vi "SPD.Insens Meas Insens_Grid.vi"(5 "Continue":refnum<vi>, 6 "deadtime index":i32, 7 "Progress":refnum<vi>, 8 "Error In":errorcluster, 11 "SPD.Stand Ctrl in":T2={"spdDeviceSession"={"spdRef"=0, "connected"=FALSE, "spdName"="", "specification"={"diod case"=enum."default", "type"=enum."Unknown", "frequency"=enum."Unknown"}, "hidSPD.Controller"={"TSet"=0.0, "HV_bias"=0.0, "DDS_stb_code"=0}, "hidSPD.Sturtup Values"={"TSet"=0.0, "HV_bias"=0.0, "DDS_stb_code"=0}}, "DevBSession"={"DevBRef"="", "connected"=FALSE}, "FreqCSession"={"FreqCRef"="", "timeout"=0.0, "Gate"=0.0, "connected"=FALSE}, "8164BSession"={"Connection ID"=refnum, "Connected"=FALSE, "Info"="", "Slots Info"=[]}, "LeCroySession"={"LeCroySession"="", "connected"=FALSE}, "Events"={"DCRTest"=refnum, "Stop"=refnum}, "configFile"={"configFile ref"=refnum, "configFile path"=path "", "equipmentFile ref"=refnum}, "SPD.Meas Grid"={"DateTime"="", "DT"=[], "Insensitivity"=[], "Temprature"=[], "Stb_code"=[], "HV_Bias"=[]}, "SPD.Queues"={"state queue"=refnum}, "Console"=refnum} {"spdDeviceSession"."hidSPD.Sturtup Values"."HV_bias" format="%#_6p, V"; "spdDeviceSession"."hidSPD.Sturtup Values"."TSet" format="%#_6p, DegC"; "spdDeviceSession"."hidSPD.Controller"."HV_bias" format="%#_6p, V"; "spdDeviceSession"."hidSPD.Controller"."TSet" format="%#_6p, DegC"}) -> (0 "Error Out":errorcluster, 1 "pass":bool, 2 "Report":string, 3 "SPD.Stand Ctrl out":T2={"spdDeviceSession"={"spdRef"=0, "connected"=FALSE, "spdName"="", "specification"={"diod case"=enum."default", "type"=enum."Unknown", "frequency"=enum."Unknown"}, "hidSPD.Controller"={"TSet"=0.0, "HV_bias"=0.0, "DDS_stb_code"=0}, "hidSPD.Sturtup Values"={"TSet"=0.0, "HV_bias"=0.0, "DDS_stb_code"=0}}, "DevBSession"={"DevBRef"="", "connected"=FALSE}, "FreqCSession"={"FreqCRef"="", "timeout"=0.0, "Gate"=0.0, "connected"=FALSE}, "8164BSession"={"Connection ID"=refnum, "Connected"=FALSE, "Info"="", "Slots Info"=[]}, "LeCroySession"={"LeCroySession"="", "connected"=FALSE}, "Events"={"DCRTest"=refnum, "Stop"=refnum}, "configFile"={"configFile ref"=refnum, "configFile path"=path "", "equipmentFile ref"=refnum}, "SPD.Meas Grid"={"DateTime"="", "DT"=[], "Insensitivity"=[], "Temprature"=[], "Stb_code"=[], "HV_Bias"=[]}, "SPD.Queues"={"state queue"=refnum}, "Console"=refnum} {"spdDeviceSession"."hidSPD.Sturtup Values"."HV_bias" format="%#_6p, V"; "spdDeviceSession"."hidSPD.Sturtup Values"."TSet" format="%#_6p, DegC"; "spdDeviceSession"."hidSPD.Controller"."HV_bias" format="%#_6p, V"; "spdDeviceSession"."hidSPD.Controller"."TSet" format="%#_6p, DegC"})   [LabVIEW 2018]
uses:
  typedefs/SPD.Stand Ctrl.ctl
  Instruments/SPD HID Interface/hidSPDLibForLabView/LibVIs/hidSPD Controls/hidSPD Device Session.ctl
  Instruments/SPD HID Interface/hidSPDLibForLabView/LibVIs/hidSPD Controls/hidSPD.SPD specification.ctl
  Instruments/SPD HID Interface/hidSPDLibForLabView/LibVIs/hidSPD Controls/hidSPD SPD Diod Case.ctl
  Instruments/SPD HID Interface/hidSPDLibForLabView/LibVIs/hidSPD Controls/hidSPD SPD Type.ctl
  Instruments/SPD HID Interface/hidSPDLibForLabView/LibVIs/hidSPD Controls/hidSPD.STB Frequency.ctl
  Instruments/SPD HID Interface/hidSPDLibForLabView/LibVIs/hidSPD Controls/hidSPD Controller.ctl
  Instruments/KC705 DevBoard/typedefs/DevB.Session.ctl
  Instruments/KeySight 53230A/typedefs/FreqC.Session.ctl
  Instruments/KeySight 8164B/KeySight 8164B LAN InstrLib/typedefs/KeySight 8164B control.ctl
  Instruments/LeCroy SDA830/typedefs/LeCroy.Session.ctl
  typedefs/SPD.Events.ctl
  ConfigFile/SPD.Config File ctrl.ctl
  <vilib>/Utility/config.llb/Config Data RefNum.ctl
  typedefs/SPD.Meas Grid.ctl
  typedefs/SPD.Queues.ctl
  typedefs/SPD.Stand state.ctl
  typedefs/SPD.Common HW Setup ctr.ctl
  typedefs/SPD.QE Strobe_Phase Tune Limits.ctl
  <vilib>/Analysis/1siggen.llb/Ramp Pattern by Delta.vi
  <vilib>/Analysis/NI_AALBase.lvlib
  Instruments/KeySight 8164B/KeySight 8164B LAN InstrLib.lvlib
  <vilib>/Utility/config.llb/NI_LVConfig.lvlib
  Instruments/SPD HID Interface/hidSPDLibForLabView/hidSPDLibForLabView.lvlib
panel:
  out "XY Graph":T1(graph)
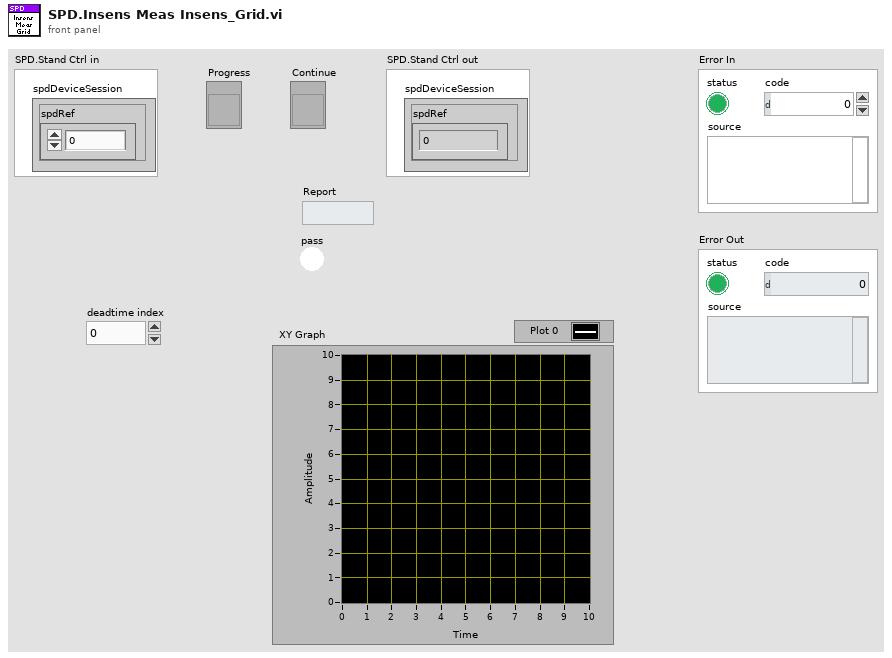
[diagram p1: front panel]
types:
  T1 = cluster{"result out":dbl[], "result out":dbl[]}[]
  T2 = typedef "SPD.Stand Ctrl.ctl" = cluster{"spdDeviceSession":T3, "DevBSession":T9, "FreqCSession":T10, "8164BSession":T11, "LeCroySession":T12, "Events":T13, "configFile":T14, "SPD.Meas Grid":T16, "SPD.Queues":T17, "Console":refnum<vi>}
  T3 = typedef "hidSPDLibForLabView.lvlib/hidSPD Device Session.ctl" = cluster{"spdRef":u64, "connected":bool, "spdName":string, "specification":T4, "hidSPD.Controller":T8, "hidSPD.Sturtup Values":T8}
  T4 = typedef "hidSPDLibForLabView.lvlib/hidSPD.SPD specification.ctl" = cluster{"diod case":T5, "type":T6, "frequency":T7}
  T5 = typedef "hidSPDLibForLabView.lvlib/hidSPD SPD Diod Case.ctl" = enum16{"Unknown", "default", "butterfly"}
  T6 = typedef "hidSPDLibForLabView.lvlib/hidSPD SPD Type.ctl" = enum16{"Unknown", "Free Run", "Gate"}
  T7 = typedef "hidSPDLibForLabView.lvlib/hidSPD.STB Frequency.ctl" = enum16{"Unknown", "312", "1250"}
  T8 = typedef "hidSPDLibForLabView.lvlib/hidSPD Controller.ctl" = cluster{"TSet":sgl, "HV_bias":sgl, "DDS_stb_code":u16}
  T9 = typedef "DevB.Session.ctl" = cluster{"DevBRef":refnum<visa-resource-name>, "connected":bool}
  T10 = typedef "FreqC.Session.ctl" = cluster{"FreqCRef":refnum<visa-resource-name>, "timeout":dbl, "Gate":dbl, "connected":bool}
  T11 = typedef "KeySight 8164B LAN InstrLib.lvlib/KeySight 8164B control.ctl" = cluster{"Connection ID":refnum<k5>, "Connected":bool, "Info":string, "Slots Info":string[]}
  T12 = typedef "LeCroy.Session.ctl" = cluster{"LeCroySession":refnum<visa-resource-name>, "connected":bool}
  T13 = typedef "SPD.Events.ctl" = cluster{"DCRTest":refnum<user-event>, "Stop":refnum<user-event>}
  T14 = typedef "SPD.Config File ctrl.ctl" = cluster{"configFile ref":T15, "configFile path":path, "equipmentFile ref":T15}
  T15 = typedef "NI_LVConfig.lvlib/Config Data RefNum.ctl" = refnum<k1>
  T16 = typedef "SPD.Meas Grid.ctl" = cluster{"DateTime":string, "DT":dbl[], "Insensitivity":dbl[], "Temprature":dbl[], "Stb_code":dbl[], "HV_Bias":dbl[][][][]}
  T17 = typedef "SPD.Queues.ctl" = cluster{"state queue":refnum<queue>}
  T18 = typedef "SPD.Common HW Setup ctr.ctl" = cluster{"FS":i32, "TS":i32, "Gate":dbl, "Att1 enable":bool, "Att3 enable":bool, "Att3 Att":dbl, "Scope setup file path":string, "Pset":dbl, "Set Pset":bool}
  T19 = typedef "SPD.DT&Insens Test Params.ctl" = cluster{"FS":i32, "TS":i32, "Att3":dbl, "Gate":dbl, "Num of Meas":i32, "ScopeRecallFile":string, "HistoSize":i32, "DT_min":u16, "DT_max":u16, "DT_step":u16, "Desired_DTs":dbl[], "Insens_bound":u16, "Insens_step":u16}
  T20 = typedef "SPD.QE Strobe_Phase Tune Limits.ctl" = cluster{"ph_start":i32, "ph_stop":i32, "ph_step":i32}
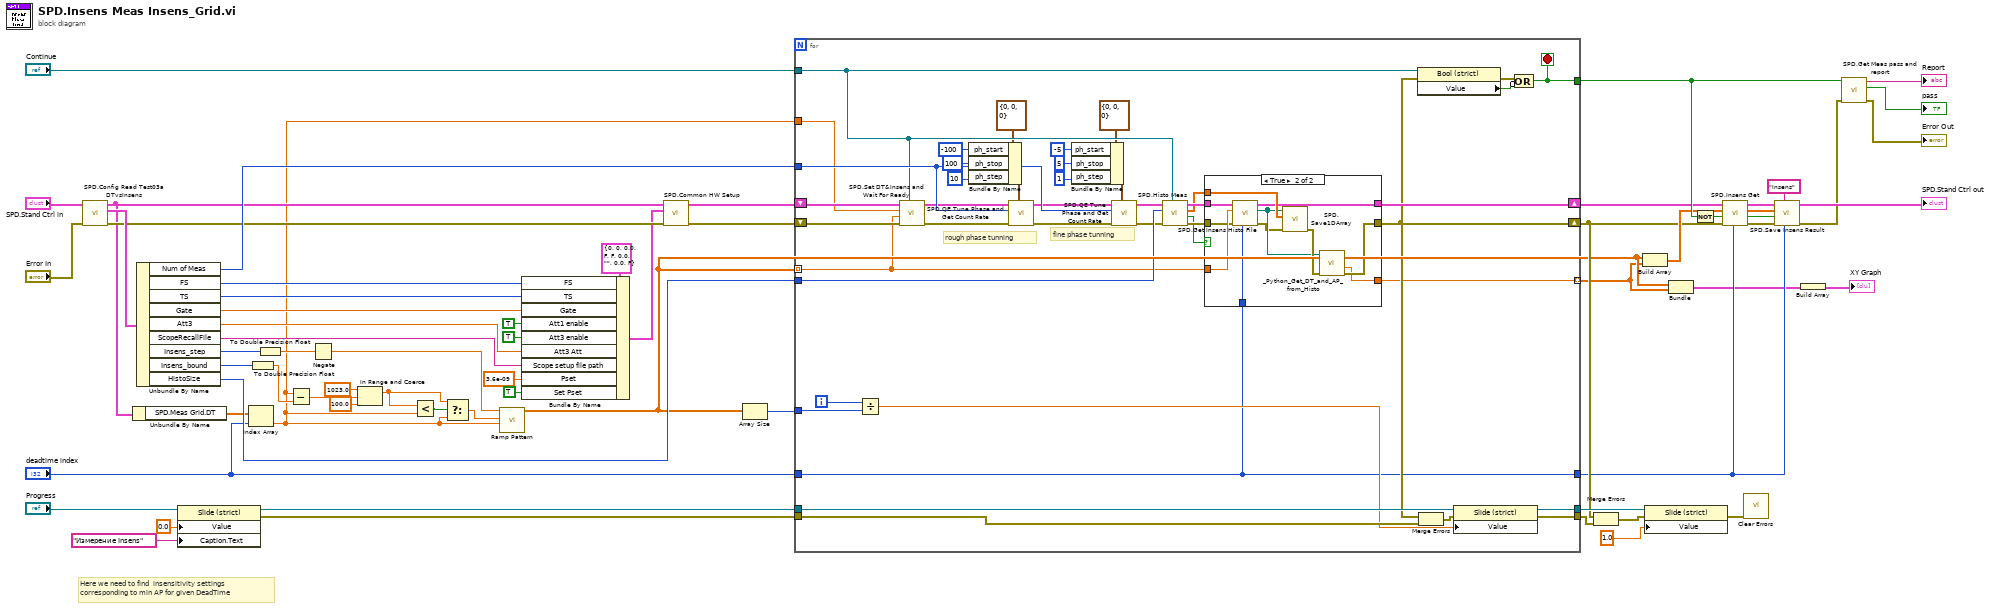
[diagram p0: block diagram]
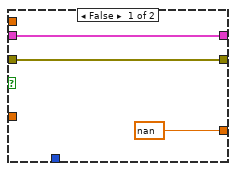
[diagram p2: hidden frame]
diagram:
  # "Here we need to find  insensitivity settings \ncorresponding to min AP for given DeadTime"
  n1 = call "SPD.Config Read Test03a DTvsInsens.vi"("Error In"="Error In", "SPD.Stand Ctrl in"="SPD.Stand Ctrl in") -> ("Error Out"=w44:errorcluster, "DTvsInsens Params"=w45:T19, "SPD.Stand Ctrl out"=w23:T2)  [unwired: 7 in]
  n2 = Unbundle By Name(w23) -> ("SPD.Meas Grid.DT"=w22:dbl[])
  n3 = Unbundle By Name(w45) -> ("Num of Meas"=w62:i32, "FS"=w51:i32, "TS"=w50:i32, "Gate"=w42:dbl, "Att3"=w41:dbl, "ScopeRecallFile"=w40:string, "Insens_step"=w31:u16, "Insens_bound"=w30:u16, "HistoSize"=w36:i32)
  n4 = property class="Slide (strict)"(reference="Progress", "Value"=0.0, "Caption.Text"="Измерение Insens") -> (reference out=w58:refnum<vi>, error out=w56:errorcluster)  [unwired: 1 in]
  n5 = Index Array(array=w22, index="deadtime index") -> (element=w2:dbl)
  n6 = To Double Precision Float(number=w30) -> (double precision float=w27:dbl)
  n7 = To Double Precision Float(number=w31) -> (double precision float=w28:dbl)
  n8 = Subtract(x=w2, y=w27) -> (x-y=w26:dbl)
  n9 = Negate(x=w28) -> (-x=w29:dbl)
  n10 = In Range and Coerce(upper limit=1023.0, x=w26, lower limit=100.0) -> (coerced(x)=w3:dbl)  [unwired: 1 out]
  n11 = Less?(x=w3, y=w2) -> (x < y?=w4:bool)
  n12 = Select(t=w3, s=w4, f=w2) -> (s? t:f=w1:dbl)
  n13 = call-poly <vilib>:"Ramp Pattern.vi"("start"=w2, "end"=w1, "delta"=w29) -> ("Ramp Pattern"=w7:dbl[])  [unwired: 6 in, 2 out]
  n14 = Bundle By Name(cluster=T18 {"FS"=0, "TS"=0, "Gate"=0.0, "Att1 enable"=FALSE, "Att3 enable"=FALSE, "Att3 Att"=0.0, "Scope setup file path"="", "Pset"=0.0, "Set Pset"=FALSE} ("common hw setup"), "FS"=w51, "TS"=w50, "Gate"=w42, "Att1 enable"=TRUE, "Att3 enable"=TRUE, "Att3 Att"=w41, "Scope setup file path"=w40, "Pset"=3.6e-09, "Set Pset"=TRUE) -> (w43:T18)
  n15 = call "SPD.Common HW Setup.vi"("error in (no error)"=w44, "common hw setup"=w43, "SPD.Stand Ctrl in in"=w23) -> ("error out"=w34:errorcluster, "SPD.Stand Ctrl out"=w33:T2)  [unwired: 7 in]
  n16 = Array Size(array=w7) -> (size(s)=w37:i32)
  n17 = for {
    shift-right: [w108] -> w17
    shift-left: w33 -> [w101]
    shift-right: [w92] -> w15
    shift-left: w34 -> [w100]
    tunnel: "Continue" -> [w99]
    tunnel: [w107] -> w35
    tunnel: w58 -> [w106]
    tunnel: [w105] -> w65
    tunnel: w62 -> [w104]
    tunnel: w56 -> [w103]
    tunnel: [w102] -> w54
    tunnel: w7 -> [w68] mode=indexing
    tunnel: w37 -> [w90]
    tunnel: w36 -> [w93]
    tunnel: w2 -> [w89]
    tunnel: "deadtime index" -> [w67]
    tunnel: [w67] -> w13
    tunnel: [w91] -> w6 mode=indexing
    i -> [w94]
    stop <- w107 stop-if-true
    # "fine phase tunning"
    # "rough phase tunning"
    n18 = Divide(x=w94, y=w90) -> (x/y=w96:dbl)
    n19 = call "SPD.Set DT&Insens and Wait For Ready.vi"("Continue"=w99, "Error In"=w100, "insensitivity"=w68, "deadtime"=w89, "SPD.Stand Ctrl in"=w101) -> ("Error Out"=w87:errorcluster, "SPD.Stand Ctrl out"=w88:T2)  [unwired: 5 in]
    n20 = Bundle By Name(cluster=T20 {"ph_start"=0, "ph_stop"=0, "ph_step"=0} ("SPD.QE Strobe_Phase Tune Limits"), "ph_start"=-100, "ph_stop"=100, "ph_step"=10) -> (w71:T20)
    n21 = call "SPD.QE Tune Phase and Get Count Rate.vi"("SPD.QE Strobe_Phase Tune Limits"=w71, "Error In"=w87, "Num of FreqC Meas"=w104, "SPD.Stand Ctrl in"=w88) -> ("Error Out"=w76:errorcluster, "SPD.Stand Ctrl out"=w77:T2)  [unwired: 4 in, 2 out]
    n22 = Bundle By Name(cluster=T20 {"ph_start"=0, "ph_stop"=0, "ph_step"=0} ("SPD.QE Strobe_Phase Tune Limits"), "ph_start"=-5, "ph_stop"=5, "ph_step"=1) -> (w81:T20)
    n23 = call "SPD.QE Tune Phase and Get Count Rate.vi"("SPD.QE Strobe_Phase Tune Limits"=w81, "Error In"=w76, "Num of FreqC Meas"=w104, "SPD.Stand Ctrl in"=w77) -> ("Error Out"=w69:errorcluster, "SPD.Stand Ctrl out"=w70:T2)  [unwired: 4 in, 2 out]
    n24 = call "SPD.Histo Meas.vi"("Continue"=w99, "Error In"=w69, "Histo length"=w93, "SPD.Stand Ctrl in"=w70) -> ("Error Out"=w84:errorcluster, "pass"=w83:bool, "Histo"=w85:dbl[], "SPD.Stand Ctrl out"=w86:T2)  [unwired: 4 in]
    n25 = case shown="True" w83 {
      tunnel: [w111 w118] -> w108
      tunnel: [w110 w120] -> w92
      tunnel: w86 -> [w111 w119]
      tunnel: w85 -> [_ w122]
      tunnel: w84 -> [w110 w116]
      tunnel: [nan ("After Pulse") w112] -> w91
      tunnel: w67 -> [_ w113]
      tunnel: w68 -> [_ w117]
      frame False {
      }
      frame True {
        n26 = call "SPD.Get Insens Histo File.vi"("DT index"=w113, "Error In"=w116, "Insens"=w117, "SPD.Stand Ctrl in"=w119) -> ("Error Out"=w114:errorcluster, "DT Results path"=w115:path, "SPD.Stand Ctrl out"=w118:T2)  [unwired: 5 in]
        n27 = call "SPD.Save1DArray.vi"("Error In"=w114, "Array"=w122, "File Path"=w115) -> ("Error Out"=w121:errorcluster)  [unwired: 8 in]
        n28 = call "_Python_Get_DT_and_AP_from_Histo.vi"("error in (no error)"=w121, "Histo path"=w115) -> ("error out"=w120:errorcluster, "After Pulse"=w112:dbl)  [unwired: 7 in, 1 out]
      }
    }
    n29 = property class="Bool (strict)"(reference=w99, error in=w92) -> (error out=w97:errorcluster, "Value"=w98:bool)  [unwired: 1 out]
    n30 = Merge Errors(w92, w103) -> (w95:errorcluster)
    n31 = property class="Slide (strict)"(reference=w106, error in=w95, "Value"=w96) -> (reference out=w105:refnum<vi>, error out=w102:errorcluster)
    n32 = Compound Arithmetic op=OR(w97, invert w98) -> (w107:bool)
  }
  n33 = Merge Errors(w15, w54) -> (w55:errorcluster)
  n34 = Build Array(w7, w6) -> (w16:dbl[][])
  n35 = property class="Slide (strict)"(reference=w65, error in=w55, "Value"=1.0) -> (error out=w63:errorcluster)  [unwired: 1 out]
  n36 = Bundle("Ramp Pattern"=w7, w6) -> (w5:cluster{"Ramp Pattern":dbl[], dbl[]})  [unwired: 1 in]
  n37 = Not(x=w35) -> (.not. x?=w14:bool)
  n38 = call "SPD.Insens Get.vi"("deadtime index"=w13, "Error In"=w15, "valid in"=w14, "Result"=w16, "SPD.Stand Ctrl in"=w17) -> ("Error Out"=w12:errorcluster, "valid out"=w11:bool, "result out"=w10:dbl[][], "SPD.Stand Ctrl out"=w9:T2)  [unwired: 3 in]
  n39 = call <vilib>:"Clear Errors.vi"("error in (no error)"=w63) -> ()  [unwired: 5 in, 2 out]
  n40 = call "SPD.Save Insens Result.vi"("DT index"=w13, "Name"="Insens", "Error In"=w12, "write to file"=w11, "Result"=w10, "SPD.Stand Ctrl in"=w9) -> ("Error Out"=w18:errorcluster, "SPD.Stand Ctrl out"=→"SPD.Stand Ctrl out":T2)  [unwired: 4 in]
  n41 = Build Array(w5) -> (→"XY Graph":cluster{"Ramp Pattern":dbl[], dbl[]}[])
  n42 = call "SPD.Get Meas pass and report.vi"("error in (no error)"=w18, "error or stoped"=w35) -> ("error out"=→"Error Out":errorcluster, "pass"=→"pass":bool, "report"=→"Report":string)  [unwired: 7 in]
